vi "Generate sorted scan parameters.vi"(1 "Array":T1(array[cluster]) {"Ramp Cluster"."phase (deg)" format="%#.4p"; "Ramp Cluster"."cycles (1,2,...)" min=1; "Ramp Cluster"."step size" format="%#.4p"; "Ramp Cluster"."Min" format="%#_6p"; "Ramp Cluster"."Max" format="%#_6p"}) -> (0 "Sorted Array":T1(array[cluster]) {"Ramp Cluster"."phase (deg)" format="%#.4p"; "Ramp Cluster"."cycles (1,2,...)" min=1; "Ramp Cluster"."step size" format="%#.4p"; "Ramp Cluster"."Min" format="%#_6p"; "Ramp Cluster"."Max" format="%#_6p"})   [LabVIEW 2011]
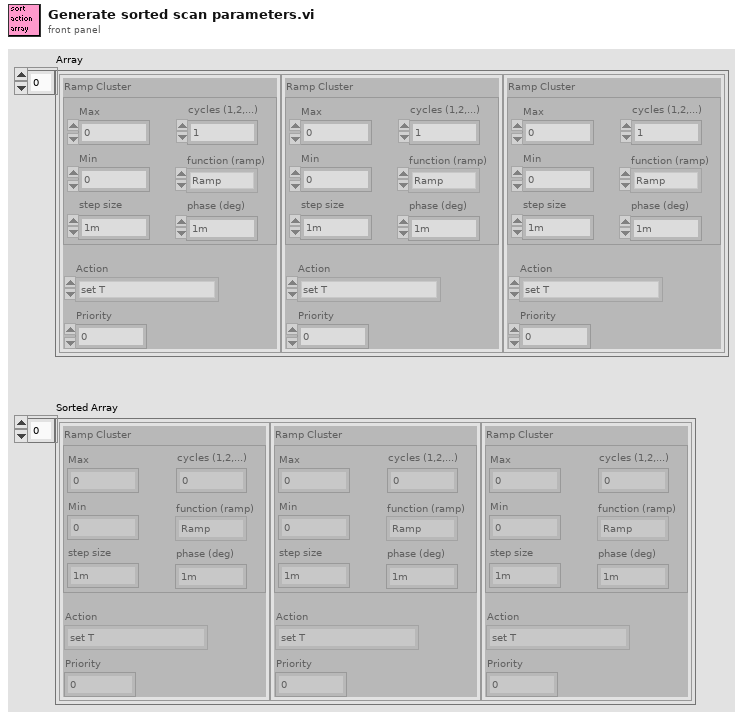
[diagram p1: front panel]
types:
  T1 = cluster{"Ramp Cluster":cluster{"Max":dbl, "Min":dbl, "step size":dbl, "cycles (1,2,...)":i32, "phase (deg)":dbl, "function (ramp)":enum16{"Ramp", "Triangle", "Sine"}}, "Action":enum16{"set T", "set B", "set Vsg1", "set Vsg2", "set lockin DC offset"}, "Priority":i32}[]
  T2 = cluster{"Ramp Cluster":cluster{"Max":dbl, "Min":dbl, "step size":dbl, "cycles (1,2,...)":i32, "phase (deg)":dbl, "function (ramp)":enum16{"Ramp", "Triangle", "Sine"}}, "Action":enum16{"set T", "set B", "set Vsg1", "set Vsg2", "set lockin DC offset"}, "Priority":i32}
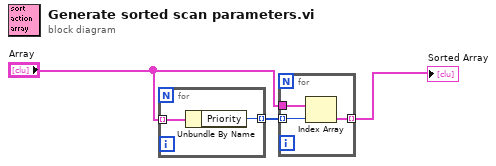
[diagram p0: block diagram]
diagram:
  n1 = for {
    tunnel: "Array" -> [w5] mode=indexing
    tunnel: [w4] -> w3 mode=indexing
    n2 = Unbundle By Name(w5) -> ("Priority"=w4:i32)
  }
  n3 = for {
    tunnel: "Array" -> [w8]
    tunnel: w3 -> [w7] mode=indexing
    tunnel: [w6] -> w2 mode=indexing
    n4 = Index Array(array=w8, index=w7) -> (element=w6:T2)
  }
  "Sorted Array" <- w2
